vi "Get ControlValue (bool).vi"(8 "Error In":errorcluster caption="エラー入力", 10 "Control Name":string, 11 "VI refnum in":refnum<vi>) -> (0 "Error Out":errorcluster caption="エラー出力", 2 "Value":bool, 3 "VI refnum out":refnum<vi>)   [LabVIEW 2018]
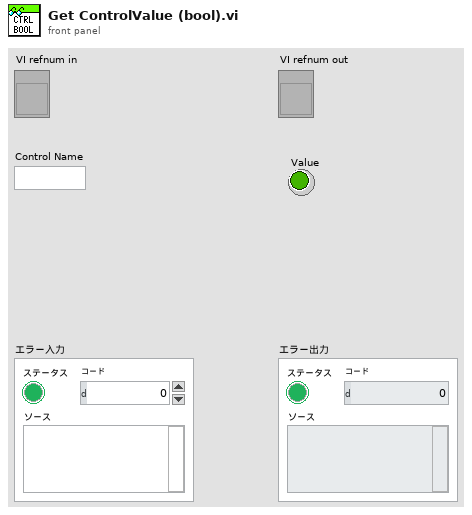
[diagram p1: front panel]
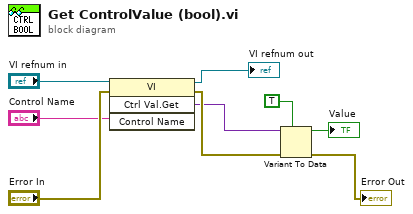
[diagram p0: block diagram]
diagram:
  n1 = invoke class="VI" method="Ctrl Val.Get"(reference="VI refnum in", error in="Error In", "Control Name"="Control Name") -> (reference out=→"VI refnum out":refnum<vi>, error out=w5:errorcluster, "Get Control Value Variant"=w3:variant)  [unwired: 1 in, 1 out]
  n2 = Variant To Data(error in=w5, type=TRUE, Variant=w3) -> (data=→"Value":bool, error out=→"Error Out":errorcluster)
